vi "UpdateUI.vi"(8 "error in":errorcluster, 9 "Control Data":variant, 10 "Action":string, 11 "UI_Manager in":refnum<class "UI_Library.lvclass">) -> (0 "error out":errorcluster, 3 "UI_Manager out":refnum<class "UI_Library.lvclass">)   [LabVIEW 2018, in "UI_Library.lvlib" / "UI_Library.lvclass"]
doc: "Handle the UI messages."
uses:
  UI_Library.lvclass
  UI_Library.lvclass/UI_Library.ctl
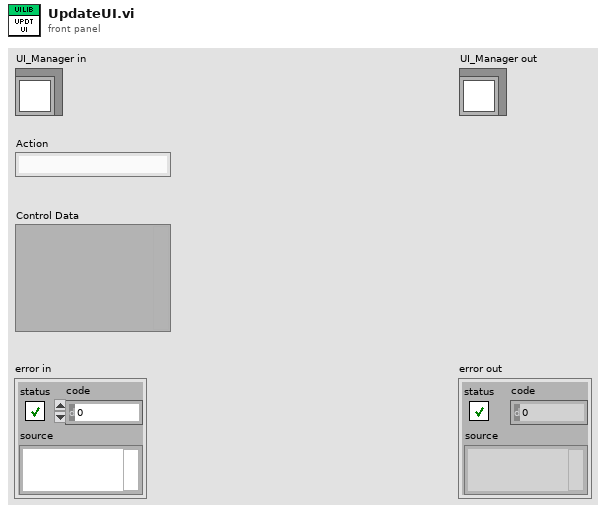
[diagram p1: front panel]
types:
  T1 = cluster{"Ctl_Refnum":refnum<vi>, "Found":bool, "Control Data":variant, "error out":errorcluster}
  T2 = enum8{"Enabled", "Disabled", "Disabled and Grayed Out"}
  T3 = typedef "UI_Library.lvlib/UI_RefCluster.ctl" = cluster{"UI Ctrl Names":string[], "UI Ctrl DataType":T4[], "UI Ctrl Refs":refnum<vi>[]}
  T4 = typedef "NI_Data Type.lvlib/Data Type.ctl" = enum8{"Invalid Type", "Void", "I8", "I16", "I32", "I64", "U8", "U16", "U32", "U64", "Single Float", "Double Float", "Extended Float", "Single Complex", "Double Complex", "Extended Complex", "Enum U8", "Enum U16", "Enum U32", "Enum U64", "Single Float With Unit", "Double Float With Unit", "Extended Float With Unit", "Single Complex with Unit", "Double Complex with Unit", "Extended Complex with Unit", "Boolean", "String", "Path", "Picture", "Tag", "Array", "Cluster", "Variant", "LV Variant", "Waveform", "Timestamp", "Digital Waveform", "Digital Data", "ExpressData", "Refnum", "External Data", "VI", "Poly VI", "LabVIEW Class Instance", "Fixed Point", "Set Collection", "Map Collection"}
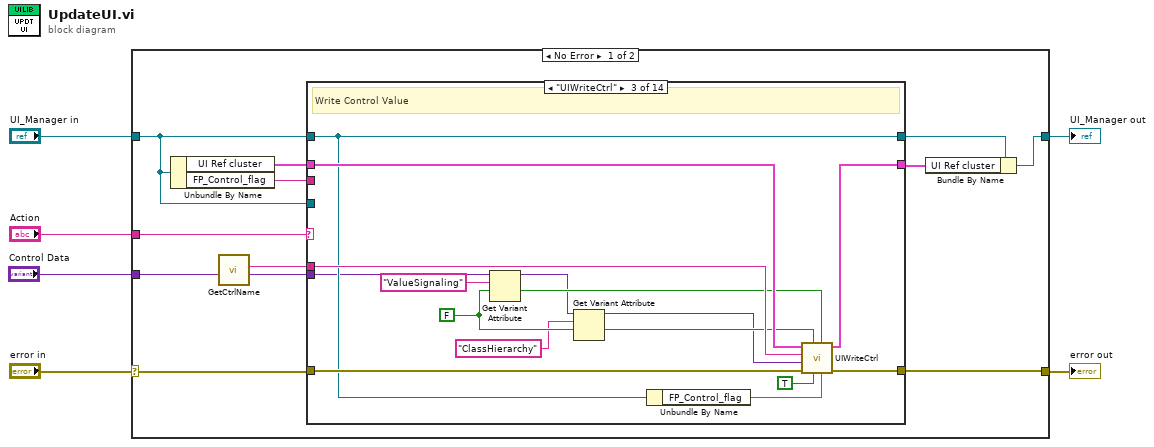
[diagram p0: block diagram]
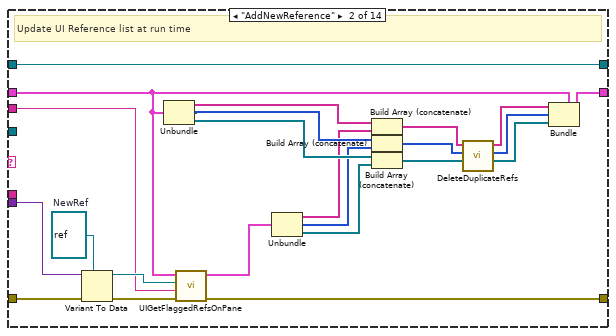
[diagram p3: hidden frame]
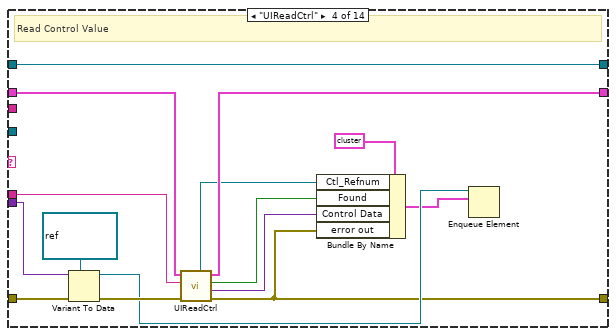
[diagram p4: hidden frame]
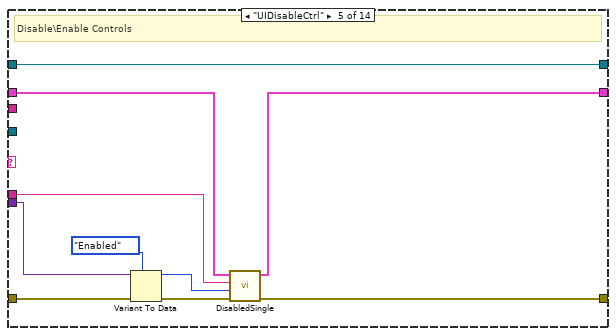
[diagram p5: hidden frame]
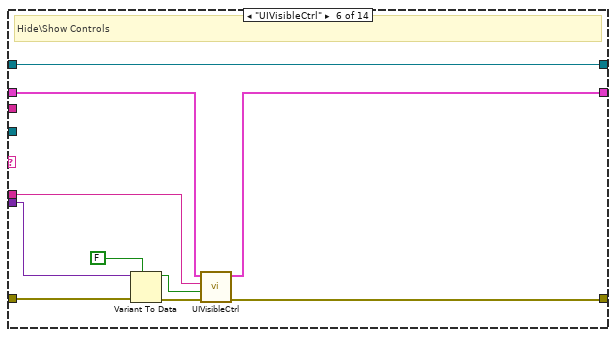
[diagram p6: hidden frame]
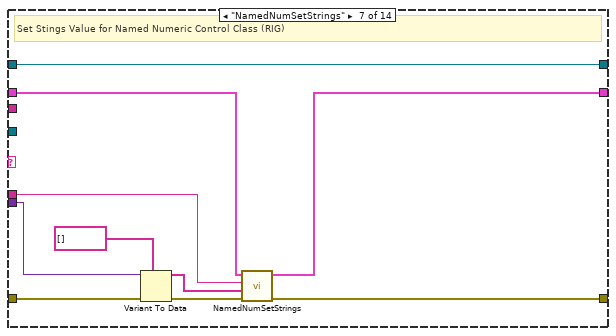
[diagram p7: hidden frame]
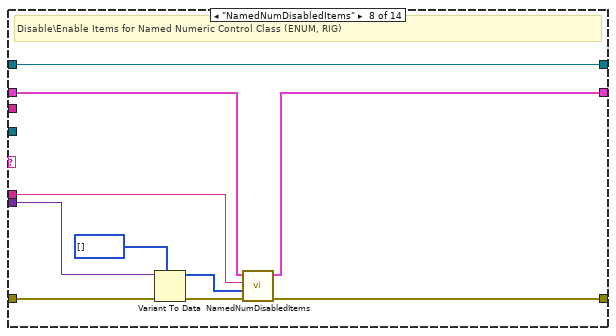
[diagram p8: hidden frame]
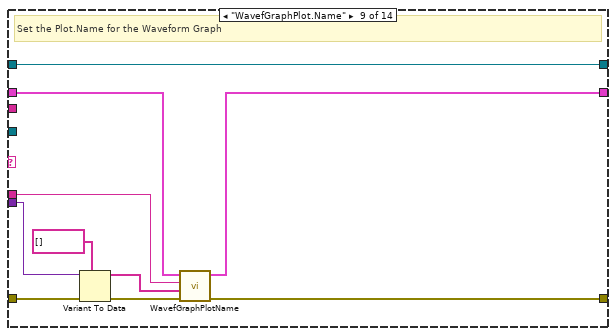
[diagram p9: hidden frame]
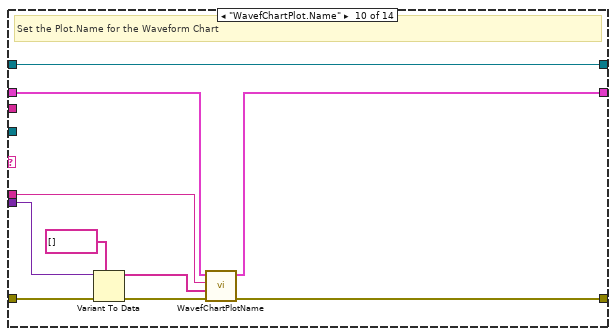
[diagram p10: hidden frame]
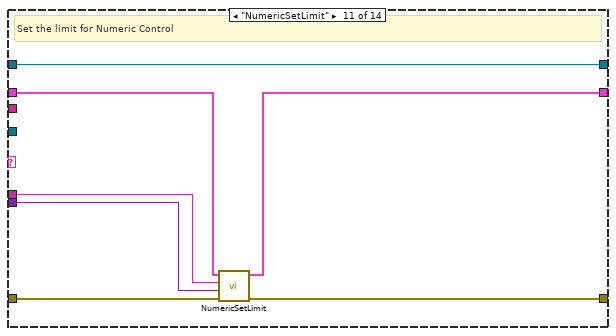
[diagram p11: hidden frame]
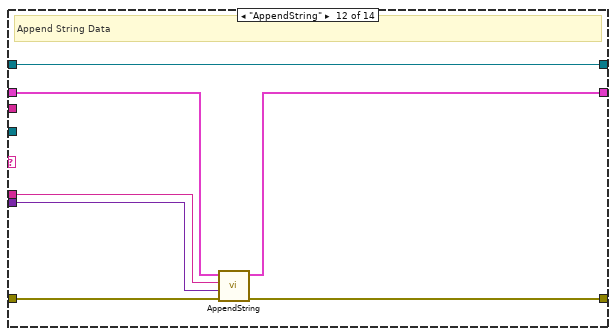
[diagram p12: hidden frame]
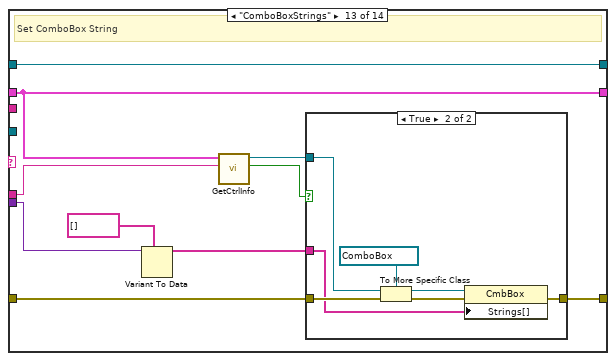
[diagram p13: hidden frame]
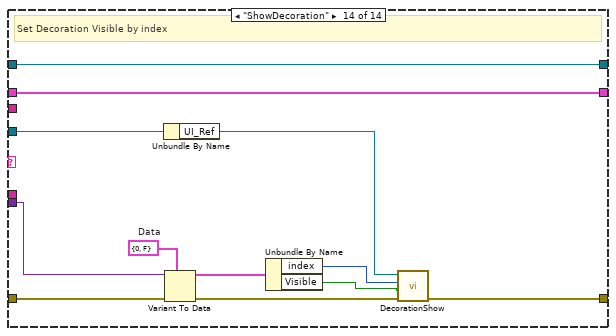
[diagram p15: hidden frame]
diagram:
  n1 = case shown="No Error" "error in" {
    selector: "error in" -> [w12 w181]
    tunnel: [w11 w181] -> w5
    tunnel: [w13 w180] -> w3
    tunnel: "UI_Manager in" -> [w8 w180]
    tunnel: "Control Data" -> [w10 _]
    tunnel: "Action" -> [w9 _]
    frame No Error {
      n2 = Unbundle By Name(w8) -> ("UI Ref cluster"=w16:T3, "FP_Control_flag"=w7:string)
      n3 = call "GetCtrlName.vi"("Control Data"=w10) -> ("Ctrl Label"=w18:string, "Data"=w17:variant)  [unwired: 5 in, 1 out]
      n4 = case shown="\"UIWriteCtrl\"" w9 {
        tunnel: w8 -> [w21 w44 w55 w75 w81 w92 w101 w111 w123 w132 w140 w146 w159 w179]
        tunnel: [w19 w40 w57 w72 w80 w91 w97 w110 w122 w131 w139 w147 w151 w177] -> w14
        tunnel: w18 -> [_ _ w59 w74 w78 w90 w100 w109 w120 w128 w138 w145 w154 _]
        tunnel: w17 -> [_ w42 w52 w70 w83 w93 w103 w113 w119 w134 w141 w144 w153 w178]
        tunnel: w12 -> [w20 w43 w60 w73 w84 w94 w104 w114 w125 w135 w142 w149 w152 w176]
        tunnel: [w20 w22 w56 w61 w79 w87 w98 w107 w121 w130 w137 w148 w150 w174] -> w11
        tunnel: w16 -> [w19 w26 w58 w67 w76 w86 w96 w106 w117 w127 w136 w143 w151 w177]
        tunnel: [w21 w44 w55 w75 w81 w92 w101 w111 w123 w132 w140 w146 w159 w179] -> w15
        tunnel: w8 -> [_ _ _ _ _ _ _ _ _ _ _ _ _ w173]
        tunnel: w7 -> [_ w25 _ _ _ _ _ _ _ _ _ _ _ _]
        frame Default {
          # "Unknow Action"
        }
        frame "AddNewReference" {
          w28 = refnum<vi> refnum  # NewRef
          # "Update UI Reference list at run time"
          n5 = Variant To Data(error in=w43, type=w28, Variant=w42) -> (data=w27:refnum<vi>, error out=w24:errorcluster)
          n6 = Unbundle(w26) -> ("UI Ctrl Names"=w41:string[], "UI Ctrl DataType"=w39:T4[], "UI Ctrl Refs"=w38:refnum<vi>[])
          n7 = call "UIGetFlaggedRefsOnPane.vi"("error in"=w24, "Flag"=w25, "VI Ref"=w27, "UI Ref cluster in"=w26) -> ("error out"=w22:errorcluster, "UI Ref cluster out"=w23:T3)  [unwired: 6 in]
          n8 = Unbundle(w23) -> ("UI Ctrl Names"=w35:string[], "UI Ctrl DataType"=w37:T4[], "UI Ctrl Refs"=w36:refnum<vi>[])
          n9 = Build Array (concatenate)(w41, w35) -> (w34:string[])
          n10 = Build Array (concatenate)(w39, w37) -> (w33:T4[])
          n11 = Build Array (concatenate)(w38, w36) -> (w32:refnum<vi>[])
          n12 = call "DeleteDuplicateRefs.vi"("CtrlRefs"=w32, "DataType"=w33, "CtrlNames"=w34) -> ("CtrlRefs out"=w29:refnum<vi>[], "DataType out"=w30:T4[], "CtrlNames out"=w31:string[])  [unwired: 6 in]
          n13 = Bundle(cluster=w26, "UI Ctrl Names"=w31, "UI Ctrl DataType"=w30, "UI Ctrl Refs"=w29) -> (w40:T3)
        }
        frame "UIWriteCtrl" {
          w48 = FALSE
          # "Write Control Value"
          n14 = Get Variant Attribute(Variant=w52, name="ValueSignaling", default value (empty Variant)=w48) -> (duplicate Variant=w46:variant, value=w50:bool)  [unwired: 1 in, 2 out]
          n15 = Get Variant Attribute(Variant=w46, name="ClassHierarchy", default value (empty Variant)=w48) -> (duplicate Variant=w45:variant, value=w49:bool)  [unwired: 1 in, 2 out]
          n16 = Unbundle By Name(w55) -> ("FP_Control_flag"=w54:string)
          n17 = call "UIWriteCtrl.vi"("UI Flag"=w54, "Value Signaling (F)"=w50, "Search Whole Word (T)"=TRUE, "Class_Hierarchy (F)"=w49, "error in"=w60, "Control Value"=w45, "Control Label"=w59, "UI Ref cluster in"=w58) -> ("error out"=w56:errorcluster, "UI Ref cluster out"=w57:T3)  [unwired: 2 in]
        }
        frame "UIReadCtrl" {
          # "Read Control Value"
          n18 = Variant To Data(error in=w73, type=refnum<queue> refnum ("queue out"), Variant=w70) -> (data=w68:refnum<queue>, error out=w71:errorcluster)
          n19 = call "UIReadCtrl.vi"("error in"=w71, "Control Label"=w74, "UI Ref cluster in"=w67) -> ("error out"=w61:errorcluster, "Control Value"=w63:variant, "Found"=w64:bool, "UI Ref cluster out"=w72:T3, "CtrlRef"=w62:refnum<vi>)  [unwired: 4 in]
          n20 = Bundle By Name(cluster=T1 {"Ctl_Refnum"=refnum, "Found"=FALSE, "Control Data"=variant, "error out"={"status"=FALSE, "code"=0, "source"=""}}, "Ctl_Refnum"=w62, "Found"=w64, "Control Data"=w63, "error out"=w61) -> (w65:T1)
          n21 = Enqueue Element(queue=w68, element=w65) -> ()  [unwired: 2 in, 3 out]
        }
        frame "UIDisableCtrl" {
          # "Disable\\Enable Controls"
          n22 = Variant To Data(error in=w84, type=T2."Enabled" ("Disabled"), Variant=w83) -> (data=w77:T2, error out=w82:errorcluster)
          n23 = call "DisabledSingle.vi"("error in"=w82, "Disabled"=w77, "Control Label"=w78, "UI Ref cluster in"=w76) -> ("error out"=w79:errorcluster, "UI Ref cluster out"=w80:T3)  [unwired: 6 in]
        }
        frame "UIVisibleCtrl" {
          # "Hide\\Show Controls"
          n24 = Variant To Data(error in=w94, type=FALSE, Variant=w93) -> (data=w88:bool, error out=w89:errorcluster)
          n25 = call "UIVisibleCtrl.vi"("error in"=w89, "Visible"=w88, "Control Label"=w90, "UI Ref cluster in"=w86) -> ("error out"=w87:errorcluster, "UI Ref cluster out"=w91:T3)  [unwired: 6 in]
        }
        frame "NamedNumSetStrings" {
          # "Set Stings Value for Named Numeric Control Class (RIG)"
          n26 = Variant To Data(error in=w104, type=string[] [], Variant=w103) -> (data=w99:string[], error out=w102:errorcluster)
          n27 = call "NamedNumSetStrings.vi"("error in"=w102, "Strings"=w99, "Control Label"=w100, "UI Ref cluster in"=w96) -> ("error out"=w98:errorcluster, "UI Ref cluster out"=w97:T3)  [unwired: 6 in]
        }
        frame "NamedNumDisabledItems" {
          # "Disable\\Enable Items for Named Numeric Control Class (ENUM, RIG)"
          n28 = Variant To Data(error in=w114, type=i32[] [], Variant=w113) -> (data=w108:i32[], error out=w112:errorcluster)
          n29 = call "NamedNumDisabledItems.vi"("error in"=w112, "Disabled Items"=w108, "Control Label"=w109, "UI Ref cluster in"=w106) -> ("error out"=w107:errorcluster, "UI Ref cluster out"=w110:T3)  [unwired: 6 in]
        }
        frame "WavefGraphPlot.Name" {
          # "Set the Plot.Name for the Waveform Graph"
          n30 = Variant To Data(error in=w125, type=string[] [], Variant=w119) -> (data=w118:string[], error out=w124:errorcluster)
          n31 = call "WavefGraphPlotName.vi"("error in"=w124, "Plot Name"=w118, "Control Label"=w120, "UI Ref cluster in"=w117) -> ("error out"=w121:errorcluster, "UI Ref cluster out"=w122:T3)  [unwired: 6 in]
        }
        frame "WavefChartPlot.Name" {
          # "Set the Plot.Name for the Waveform Chart"
          n32 = Variant To Data(error in=w135, type=string[] [], Variant=w134) -> (data=w129:string[], error out=w133:errorcluster)
          n33 = call "WavefChartPlotName.vi"("error in"=w133, "Plot Name"=w129, "Control Label"=w128, "UI Ref cluster in"=w127) -> ("error out"=w130:errorcluster, "UI Ref cluster out"=w131:T3)  [unwired: 6 in]
        }
        frame "NumericSetLimit" {
          # "Set the limit for Numeric Control"
          n34 = call "NumericSetLimit.vi"("error in"=w142, "Control Value"=w141, "Control Label"=w138, "UI Ref cluster in"=w136) -> ("error out"=w137:errorcluster, "UI Ref cluster out"=w139:T3)  [unwired: 6 in]
        }
        frame "AppendString" {
          # "Append String Data"
          n35 = call "AppendString.vi"("error in"=w149, "Control Value"=w144, "Control Label"=w145, "UI Ref cluster in"=w143) -> ("error out"=w148:errorcluster, "UI Ref cluster out"=w147:T3)  [unwired: 6 in]
        }
        frame "ComboBoxStrings" {
          # "Set ComboBox String"
          n36 = Variant To Data(type=string[] [], Variant=w153) -> (data=w156:string[])  [unwired: 1 in, 1 out]
          n37 = call "GetCtrlInfo.vi"("Ctrl Label"=w154, "UI Ref cluster"=w151) -> ("Found"=w158:bool, "Control out"=w157:refnum<vi>)  [unwired: 8 in]
          n38 = case shown="True" w158 {
            tunnel: w157 -> [_ w161]
            tunnel: w152 -> [w160 w166]
            tunnel: [w160 w167] -> w150
            tunnel: w156 -> [_ w162]
            frame False {
            }
            frame True {
              n39 = To More Specific Class(target class=refnum<vi> refnum ("reference"), reference=w161, error in=w166) -> (specific class reference=w163:refnum<vi>, error out=w165:errorcluster)
              n40 = property on="Property Node" class="CmbBox"(reference=w163, error in=w165, "Strings[]"=w162) -> (error out=w167:errorcluster)  [unwired: 1 out]
            }
          }
        }
        frame "ShowDecoration" {
          w171 = cluster{"index":i32, "Visible":bool} {"index"=0, "Visible"=FALSE}  # Data
          # "Set Decoration Visible by index"
          n41 = Unbundle By Name(w173) -> ("UI_Ref"=w172:refnum<vi>)
          n42 = Variant To Data(error in=w176, type=w171, Variant=w178) -> (data=w170:cluster{"index":i32, "Visible":bool}, error out=w175:errorcluster)
          n43 = Unbundle By Name(w170) -> ("index"=w169:i32, "Visible"=w168:bool)
          n44 = call "DecorationShow.vi"("error in (no error)"=w175, "Visible"=w168, "index"=w169, "VI_Ref"=w172) -> ("error out"=w174:errorcluster)  [unwired: 7 in]
        }
      }
      n45 = Bundle By Name(cluster=w15, "UI Ref cluster"=w14) -> (w13:refnum<class "UI_Library.lvclass">)
    }
    frame Error {
    }
  }
  "error out" <- w5
  "UI_Manager out" <- w3
